vi "array sales ex 1.vi"() -> ()   [LabVIEW 2020]
panel:
  out "col":string[](array[string])
  out "row":string[](array[string])
  in  "disabled index (col)":i32
  in  "index (row)":i32
  out "sales data":string[][](array[string])
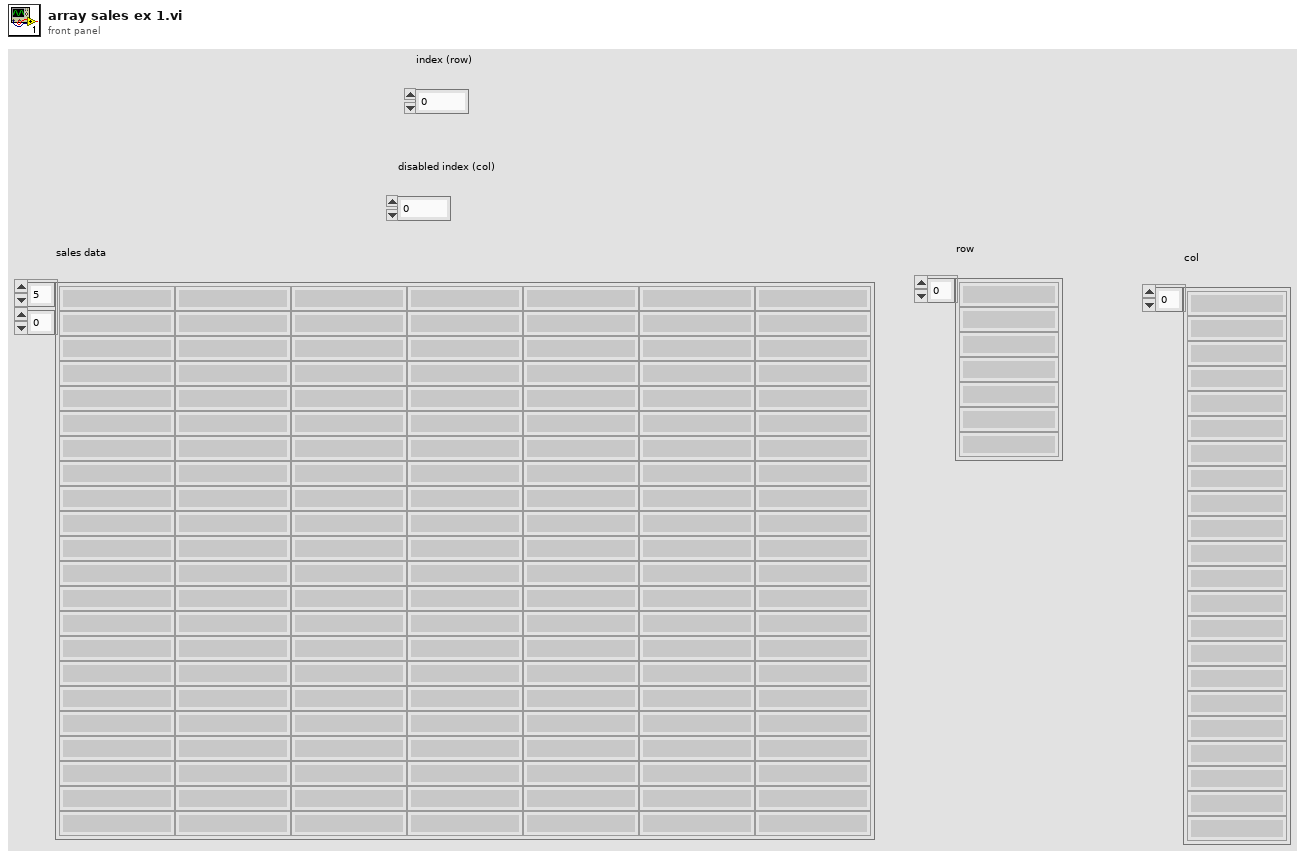
[diagram p1: front panel]
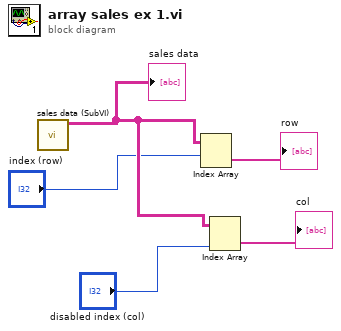
[diagram p0: block diagram]
diagram:
  n1 = call "sales data (SubVI).vi"() -> ("sales data"=w5:string[][])  [unwired: 11 in]
  "sales data" <- w5
  n2 = Index Array "Index Array"(array=w5, index (row)="index (row)") -> (element=→"row":string[])  [unwired: 1 in]
  n3 = Index Array(array=w5, index (col)="disabled index (col)") -> (element=→"col":string[])  [unwired: 1 in]
